vi "TCP Server Register Connection Handler.vi"(8 "error in (no error)":errorcluster, 10 "Connection Data":T1, 11 "RefNum":refnum<class "JKI TCP Server.lvclass">) -> (0 "error out":errorcluster, 2 "Additional Data":variant, 3 "dup RefNum":refnum<class "JKI TCP Server.lvclass">)   [LabVIEW 2020, in "JKI TCP Server.lvclass"]
uses:
  JKI TCP Server.lvclass
  _Data Structures/TCP Server Connection Process Data Cluster.ctl
  _Data Structures/TCP Server Connection Info Cluster.ctl
  JKI TCP Server.lvclass/JKI TCP Server.ctl
panel:
  # "Copyright © 2004-2008 JKI. All rights reserved.\n\nAuthor: Jim Kring [jim.kring@jameskring.com]\n\nThis library is provided \"AS IS\" ,WITHOUT WARRANTIES OR \nCONDITIONS OF ANY KIND, either express or implied.\n\nJames Kring, Inc. -- http://www.jameskring.com"
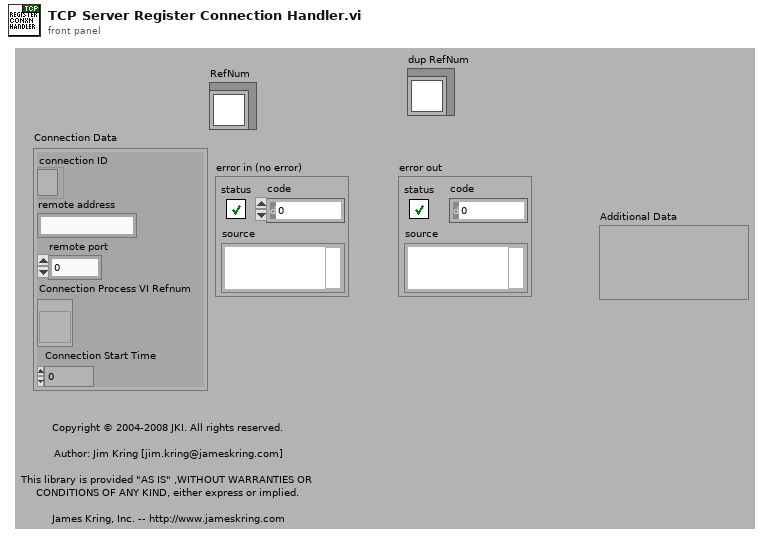
[diagram p1: front panel]
types:
  T1 = typedef "JKI TCP Server.lvclass/TCP Server Connection Process Data Cluster.ctl" = cluster{"connection ID":refnum<k5>, "remote address":string, "remote port":u16, "Connection Process VI Refnum":refnum<vi>, "Connection Start Time":u32}
  T2 = typedef "JKI TCP Server.lvclass/TCP Server Data.ctl" = cluster{"Listener Info":T3, "Connection Process VI RefNums":refnum<vi>[], "dup connection IDs (for quick search)":refnum<k5>[], "Connections":T4[], "Connection Handler VI Path":path, "Handler Is Reentrant?":bool, "TCP Handler Instance RefNums":T5[], "TCP Handler VI RefNum":T5, "No. Connections":u32, "Max Connections":u32, "server start time":u32, "Additional Data":variant}
  T3 = typedef "JKI TCP Server.lvclass/TCP Server Listener Info Cluster.ctl" = cluster{"listener ID":refnum<k5>, "net address":u32, "port":u16, "Listener Process VI Refnum":refnum<vi>}
  T4 = typedef "JKI TCP Server.lvclass/TCP Server Connection Info Cluster.ctl" = cluster{"connection ID":refnum<k5>, "Remote Address":string, "remote port":u16, "connection start time":u32}
  T5 = typedef "JKI TCP Server.lvclass/TCP Server Handler RefNum.ctl" = refnum<vi>
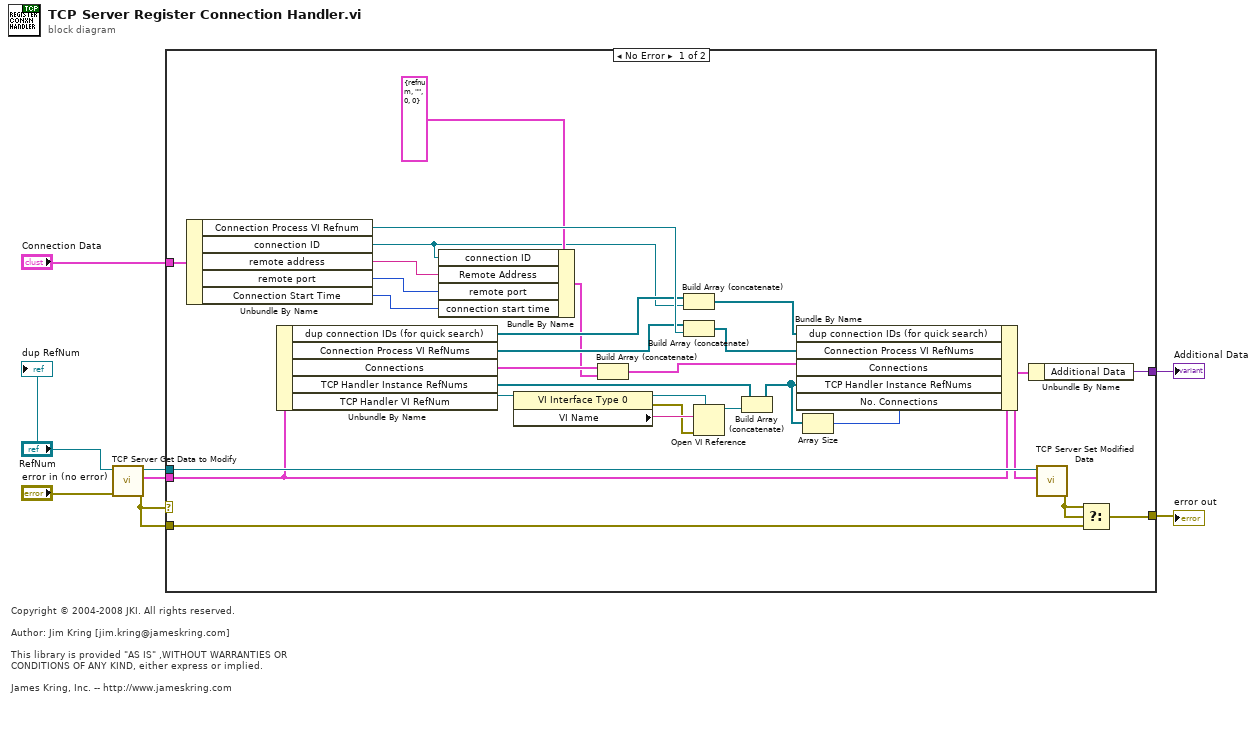
[diagram p0: block diagram]
diagram:
  # "Copyright © 2004-2008 JKI. All rights reserved.\n\nAuthor: Jim Kring [jim.kring@jameskring.com]\n\nThis library is provided \"AS IS\" ,WITHOUT WARRANTIES OR \nCONDITIONS OF ANY KIND, either express or implied.\n\nJames Kring, Inc. -- http://www.jameskring.com"
  n1 = call "TCP Server Get Data to Modify.vi"("error in (no error)"="error in (no error)", "RefNum"="RefNum") -> ("error out"=w2:errorcluster, "Data out"=w5:T2, "dup RefNum"=w6:refnum<class "JKI TCP Server.lvclass">)  [unwired: 6 in, 1 out]
  n2 = case shown="No Error" w2 {
    tunnel: "Connection Data" -> [w37 _]
    tunnel: w6 -> [w33 _]
    tunnel: w5 -> [w32 _]
    tunnel: w2 -> [w12 w38]
    tunnel: [w11 w38] -> w4
    tunnel: [w9 _] -> w1
    frame No Error {
      n3 = Unbundle By Name(w37) -> ("Connection Process VI Refnum"=w35:refnum<vi>, "connection ID"=w27:refnum<k5>, "remote address"=w26:string, "remote port"=w25:u16, "Connection Start Time"=w24:u32)
      n4 = Unbundle By Name(w32) -> ("dup connection IDs (for quick search)"=w31:refnum<k5>[], "Connection Process VI RefNums"=w34:refnum<vi>[], "Connections"=w29:T4[], "TCP Handler Instance RefNums"=w17:T5[], "TCP Handler VI RefNum"=w21:T5)
      n5 = Bundle By Name(cluster=T4 {"connection ID"=refnum, "Remote Address"="", "remote port"=0, "connection start time"=0} ("Connection Info"), "connection ID"=w27, "Remote Address"=w26, "remote port"=w25, "connection start time"=w24) -> (w23:T4)
      n6 = property class="VI Interface Type 0"(reference=w21) -> (reference out=w18:T5, error out=w19:errorcluster, "VI Name"=w20:string)  [unwired: 1 in]
      n7 = Build Array (concatenate)(w29, w23) -> (w22:T4[])
      n8 = Build Array (concatenate)(w31, w27) -> (w30:refnum<k5>[])
      n9 = Build Array (concatenate)(w34, w35) -> (w36:refnum<vi>[])
      n10 = Open VI Reference(type specifier VI Refnum (for type only)=w18, vi path=w20, error in (no error)=w19) -> (vi reference=w16:T5)  [unwired: 3 in, 1 out]
      n11 = Build Array (concatenate)(w17, w16) -> (w15:T5[])
      n12 = Array Size(array=w15) -> (size(s)=w14:i32)
      n13 = Bundle By Name(cluster=w32, "dup connection IDs (for quick search)"=w30, "Connection Process VI RefNums"=w36, "Connections"=w22, "TCP Handler Instance RefNums"=w15, "No. Connections"=w14) -> (w10:T2)
      n14 = Unbundle By Name(w10) -> ("Additional Data"=w9:variant)
      n15 = call "TCP Server Set Modified Data.vi"("Data in"=w10, "RefNum"=w33) -> ("error out"=w13:errorcluster)  [unwired: 8 in, 1 out]
      n16 = Select(t=w13, s=w13, f=w12) -> (s? t:f=w11:errorcluster)
    }
    frame Error {
    }
  }
  "error out" <- w4
  "Additional Data" <- w1
  "dup RefNum" <- "RefNum"
